vi "Deploy-Step-390-ITSERPSetup.vi"(0 "Deployment Engine":refnum<class "Deploy-DeploymentEngine.lvclass">, 11 "error in":errorcluster) -> (15 "error out":errorcluster)   [LabVIEW 2013]
uses:
  <resource>/Framework/Providers/Wirebird Labs LLC/Deploy/Support/Deployment Engine/Deploy-DeploymentEngine.lvclass
panel:
  # "Inputs"
  # "Outputs"
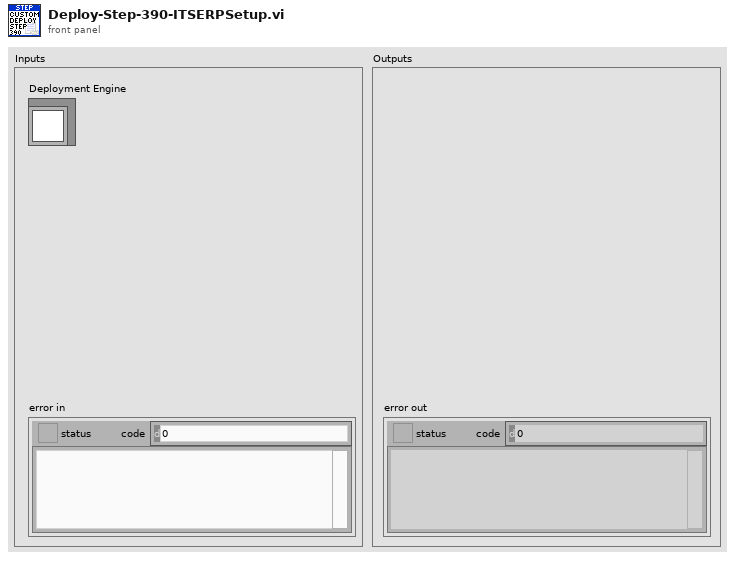
[diagram p1: front panel]
types:
  T1 = cluster{"Search for (Regular Expression)":string, "Replace with":string}[]
  T2 = typedef "Deploy-Directives-SetupFile.ctl" = cluster{"Local Filepath":path, "Root Destination Directory":T3, "Relative Destination":string, "Parameters":string}
  T3 = typedef "Deploy-InnoSetup-DirectoryConstant.ctl" = enum16{"Application Directory {app}", "Windows Directory {win}", "System32 Directory {sys}", "SysWOW64 Directory {syswow64}", "Setup Directory {src}", "Root System Drive {sd}", "Program Files {pf}", "Program Files x86 {pf32}", "Program Files x64 {pf64}", "Unique Temp Directory {tmp}", "Fonts Directory {fonts}", "Start Menu Directory {group}", "Local App Data {localappdata}", "User App Data {userappdata}", "Common App Data {commonappdata}", "SendTo Directory {sendto}", "User Common Files {usercf}", "User Desktop {userdesktop}", "Common Desktop {commondesktop}", "User Documents {userdocs}", "Common Documents {commondocs}", "User Program Files {userpf}", "User Start Menu Programs {userprograms}", "Common Start Menu Programs {commonprograms}", "User Start Menu {userstartmenu}", "Common Start Menu {commonstartmenu}", "User Startup {userstartup}", "Common Startup {commonstartup}", "User Templates {usertemplates}", "Common Templates {commontemplates}"}
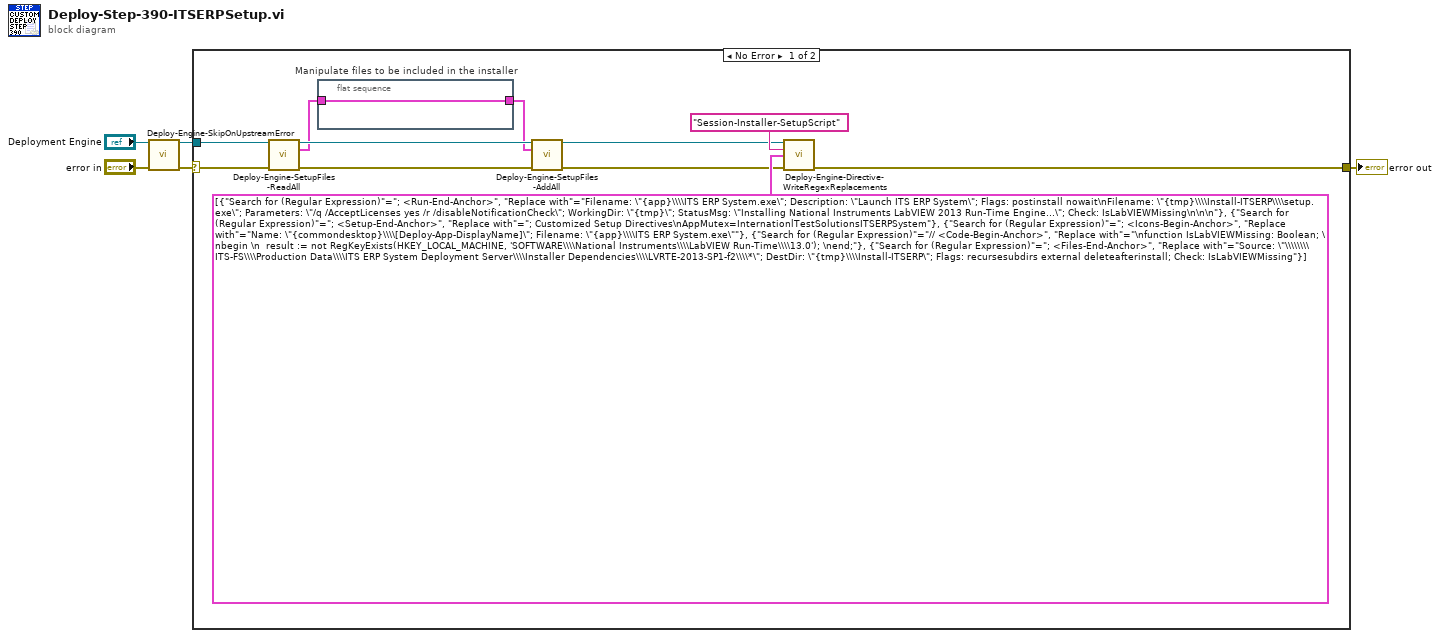
[diagram p0: block diagram]
diagram:
  n1 = call <resource>:"Deploy-Engine-SkipOnUpstreamError.vi"("Engine"="Deployment Engine", "error in"="error in") -> ("Engine out"=w2:refnum<class "Deploy-DeploymentEngine.lvclass">, "error out"=w1:errorcluster)  [unwired: 12 in]
  n2 = case shown="No Error" w1 {
    selector: w1 -> [w10 w18]
    tunnel: [w15 w18] -> w3
    tunnel: w2 -> [w11 _]
    frame No Error {
      n3 = call <resource>:"Deploy-Engine-SetupFiles-ReadAll.vi"("Engine"=w11, "error in"=w10) -> ("Engine out"=w12:refnum<class "Deploy-DeploymentEngine.lvclass">, "Setup Files"=w6:T2[], "error out"=w13:errorcluster)  [unwired: 11 in]
      n4 = flat-sequence "Manipulate files to be included in the installer" {
        tunnel: [w17] -> w7
        tunnel: w6 -> [w17]
        frame #0 {
        }
      }
      n5 = call <resource>:"Deploy-Engine-SetupFiles-AddAll.vi"("Engine"=w12, "Setup Files"=w7, "error in"=w13) -> ("Engine out"=w9:refnum<class "Deploy-DeploymentEngine.lvclass">, "error out"=w8:errorcluster)  [unwired: 11 in]
      n6 = call <resource>:"Deploy-Engine-Directive-WriteRegexReplacements.vi"("Engine"=w9, "Directive"="Session-Installer-SetupScript" ("Property Name"), "Value Replacements"=T1 [{"Search for (Regular Expression)"="; <Run-End-Anchor>", "Replace with"="Filename: \"{app}\\\\ITS ERP System.exe\"; Description: \"Launch ITS ERP System\"; Flags: postinstall nowait\nFilename: \"{tmp}\\\\Install-ITSERP\\\\setup.exe\"; Parameters: \"/q /AcceptLicenses yes /r /disableNotificationCheck\"; WorkingDir: \"{tmp}\"; StatusMsg: \"Installing National Instruments LabVIEW 2013 Run-Time Engine...\"; Check: IsLabVIEWMissing\n\n\n"}, {"Search for (Regular Expression)"="; <Setup-End-Anchor>", "Replace with"="; Customized Setup Directives\nAppMutex=InternationlTestSolutionsITSERPSystem"}, {"Search for (Regular Expression)"="; <Icons-Begin-Anchor>", "Replace with"="Name: \"{commondesktop}\\\\[Deploy-App-DisplayName]\"; Filename: \"{app}\\\\ITS ERP System.exe\""}, {"Search for (Regular Expression)"="// <Code-Begin-Anchor>", "Replace with"="\nfunction IsLabVIEWMissing: Boolean; \nbegin \n  result := not RegKeyExists(HKEY_LOCAL_MACHINE, 'SOFTWARE\\\\National Instruments\\\\LabVIEW Run-Time\\\\13.0'); \nend;"}, {"Search for (Regular Expression)"="; <Files-End-Anchor>", "Replace with"="Source: \"\\\\\\\\ITS-FS\\\\Production Data\\\\ITS ERP System Deployment Server\\\\Installer Dependencies\\\\LVRTE-2013-SP1-f2\\\\*\"; DestDir: \"{tmp}\\\\Install-ITSERP\"; Flags: recursesubdirs external deleteafterinstall; Check: IsLabVIEWMissing"}], "error in"=w8) -> ("error out"=w15:errorcluster)  [unwired: 10 in, 1 out]
    }
    frame Error {
    }
  }
  "error out" <- w3
